vi "PRO_VerifySpec.vi"(6 "error in (no error)":errorcluster, 7 "Enable":bool, 8 "Results in":T6=[[{"Fill"=0.0, "Drain"=7.150000000000002, "Status"=9, "Resistor"=100.0}, {"Fill"=0.0, "Drain"=6.925000000000003, "Status"=9, "Resistor"=100.0}], [{"Fill"=7.1350000000000025, "Drain"=6.700000000000004, "Status"=9, "Resistor"=200.0}, {"Fill"=6.910000000000004, "Drain"=6.475000000000005, "Status"=9, "Resistor"=200.0}], [{"Fill"=6.685000000000004, "Drain"=6.250000000000005, "Status"=9, "Resistor"=300.0}, {"Fill"=6.460000000000004, "Drain"=6.025000000000006, "Status"=9, "Resistor"=300.0}], [{"Fill"=6.235000000000006, "Drain"=5.8000000000000025, "Status"=9, "Resistor"=400.0}, {"Fill"=6.010000000000005, "Drain"=5.59, "Status"=9, "Resistor"=400.0}], [{"Fill"=5.785000000000002, "Drain"=5.364999999999997, "Status"=9, "Resistor"=500.0}, {"Fill"=5.574999999999999, "Drain"=5.1399999999999935, "Status"=9, "Resistor"=500.0}], [{"Fill"=5.349999999999996, "Drain"=4.91499999999999, "Status"=9, "Resistor"=600.0}, {"Fill"=5.124999999999993, "Drain"=4.689999999999987, "Status"=9, "Resistor"=600.0}], [{"Fill"=4.89999999999999, "Drain"=4.464999999999983, "Status"=9, "Resistor"=700.0}, {"Fill"=4.6749999999999865, "Drain"=4.23999999999998, "Status"=9, "Resistor"=700.0}], [{"Fill"=4.449999999999983, "Drain"=4.014999999999977, "Status"=9, "Resistor"=800.0}, {"Fill"=4.22499999999998, "Drain"=3.7899999999999734, "Status"=9, "Resistor"=800.0}], [{"Fill"=3.999999999999977, "Drain"=3.56499999999997, "Status"=9, "Resistor"=900.0}, {"Fill"=3.7749999999999737, "Drain"=3.339999999999967, "Status"=9, "Resistor"=900.0}], [{"Fill"=3.5499999999999705, "Drain"=3.114999999999964, "Status"=9, "Resistor"=1000.0}, {"Fill"=3.3249999999999673, "Drain"=2.8899999999999606, "Status"=9, "Resistor"=1000.0}], [{"Fill"=3.099999999999964, "Drain"=0.0, "Status"=5, "Resistor"=1100.0}, {"Fill"=2.874999999999961, "Drain"=0.0, "Status"=5, "Resistor"=1100.0}]] {"Resistor" format="%.1f"; "Drain" format="%.3f"; "Fill" format="%.3f"}, 9 "Measure In":T5={"Ch A   Ohms"=100.0, " Ch B  Ohms"=100.0, "Level OUt"=3.672222222222213}, 10 "Specs In":T1) -> (0 "Results out":T6=[[{"Fill"=0.0, "Drain"=7.150000000000002, "Status"=9, "Resistor"=100.0}, {"Fill"=0.0, "Drain"=6.925000000000003, "Status"=9, "Resistor"=100.0}], [{"Fill"=7.1350000000000025, "Drain"=6.700000000000004, "Status"=9, "Resistor"=200.0}, {"Fill"=6.910000000000004, "Drain"=6.475000000000005, "Status"=9, "Resistor"=200.0}], [{"Fill"=6.685000000000004, "Drain"=6.250000000000005, "Status"=9, "Resistor"=300.0}, {"Fill"=6.460000000000004, "Drain"=6.025000000000006, "Status"=9, "Resistor"=300.0}], [{"Fill"=6.235000000000006, "Drain"=5.8000000000000025, "Status"=9, "Resistor"=400.0}, {"Fill"=6.010000000000005, "Drain"=5.59, "Status"=9, "Resistor"=400.0}], [{"Fill"=5.785000000000002, "Drain"=5.364999999999997, "Status"=9, "Resistor"=500.0}, {"Fill"=5.574999999999999, "Drain"=5.1399999999999935, "Status"=9, "Resistor"=500.0}], [{"Fill"=5.349999999999996, "Drain"=4.91499999999999, "Status"=9, "Resistor"=600.0}, {"Fill"=5.124999999999993, "Drain"=4.689999999999987, "Status"=9, "Resistor"=600.0}], [{"Fill"=4.89999999999999, "Drain"=4.464999999999983, "Status"=9, "Resistor"=700.0}, {"Fill"=4.6749999999999865, "Drain"=4.23999999999998, "Status"=9, "Resistor"=700.0}], [{"Fill"=4.449999999999983, "Drain"=4.014999999999977, "Status"=9, "Resistor"=800.0}, {"Fill"=4.22499999999998, "Drain"=3.7899999999999734, "Status"=9, "Resistor"=800.0}], [{"Fill"=3.999999999999977, "Drain"=3.56499999999997, "Status"=9, "Resistor"=900.0}, {"Fill"=3.7749999999999737, "Drain"=3.339999999999967, "Status"=9, "Resistor"=900.0}], [{"Fill"=3.5499999999999705, "Drain"=3.114999999999964, "Status"=9, "Resistor"=1000.0}, {"Fill"=3.3249999999999673, "Drain"=2.8899999999999606, "Status"=9, "Resistor"=1000.0}], [{"Fill"=3.099999999999964, "Drain"=0.0, "Status"=5, "Resistor"=1100.0}, {"Fill"=2.874999999999961, "Drain"=0.0, "Status"=5, "Resistor"=1100.0}]] {"Resistor" format="%.1f"; "Drain" format="%.3f"; "Fill" format="%.3f"}, 1 "Status Code":i32, 4 "error out":errorcluster)   [LabVIEW 2024]
doc: "Compares the ChA, ChB and Level measurements to the Incexed Spec Row. Checks for R Switch Value occured in Switch Zone, The resistor level was consistand in the In Range Zone, and records the R level in ohms at the R measurement point. \n\nBuilds the Results Table."
uses:
  Control Definitions/Def Results2.ctl
  Control Definitions/DEF_SpecsOut.ctl
  Control Definitions/Ded Spec RNG.ctl
  Control Definitions/Ded LUT_Status.ctl
  Control Definitions/Def PumpCtlRefs.ctl
panel:
  # "ChA=0; ChB=1"
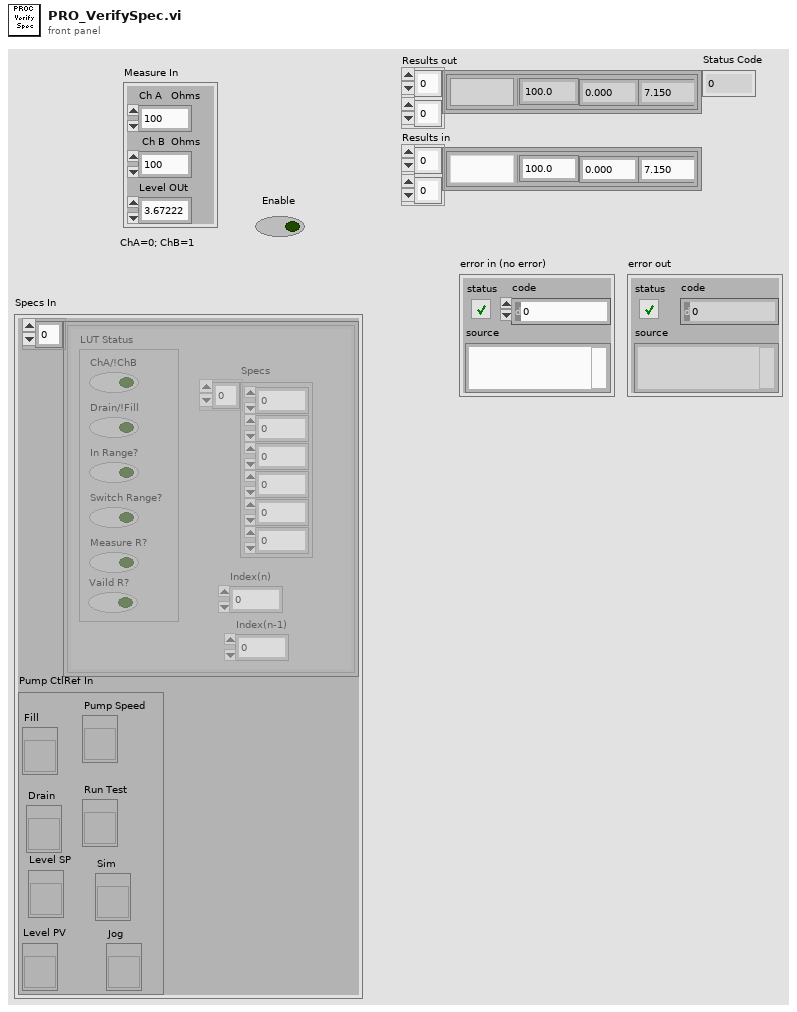
[diagram p1: front panel]
types:
  T1 = typedef "DEF_SpecsOut.ctl" = cluster{"aSpecsTable":T2[], "Pump CtlRef In":T4}
  T2 = typedef "Ded Spec RNG.ctl" = cluster{"Specs":dbl[], "Index(n)":i32, "LUT Status":T3, "Index(n-1)":i32}
  T3 = typedef "Ded LUT_Status.ctl" = cluster{"ChA/!ChB":bool, "Drain/!Fill":bool, "In Range?":bool, "Switch Range?":bool, "Measure R?":bool, "Vaild R?":bool}
  T4 = typedef "Def PumpCtlRefs.ctl" = cluster{"Fill ":refnum<vi>, "Drain":refnum<vi>, "Level PV":refnum<vi>, "Pump Speed":refnum<vi>, "Run Test":refnum<vi>, "Sim":refnum<vi>, "Jog":refnum<vi>, "Level SP":refnum<vi>}
  T5 = cluster{"Ch A   Ohms":dbl, " Ch B  Ohms":dbl, "Level OUt":dbl}
  T6 = typedef "Def Results2.ctl" = cluster{"Fill":dbl, "Drain":dbl, "Status":i16, "Resistor":dbl}[][]
  T7 = cluster{"Fill":dbl, "Drain":dbl, "Status":i16, "Resistor":dbl}
  T8 = typedef "Def_LevelSwitched.ctl" = cluster{"Switched":bool, "Level OUt":dbl}
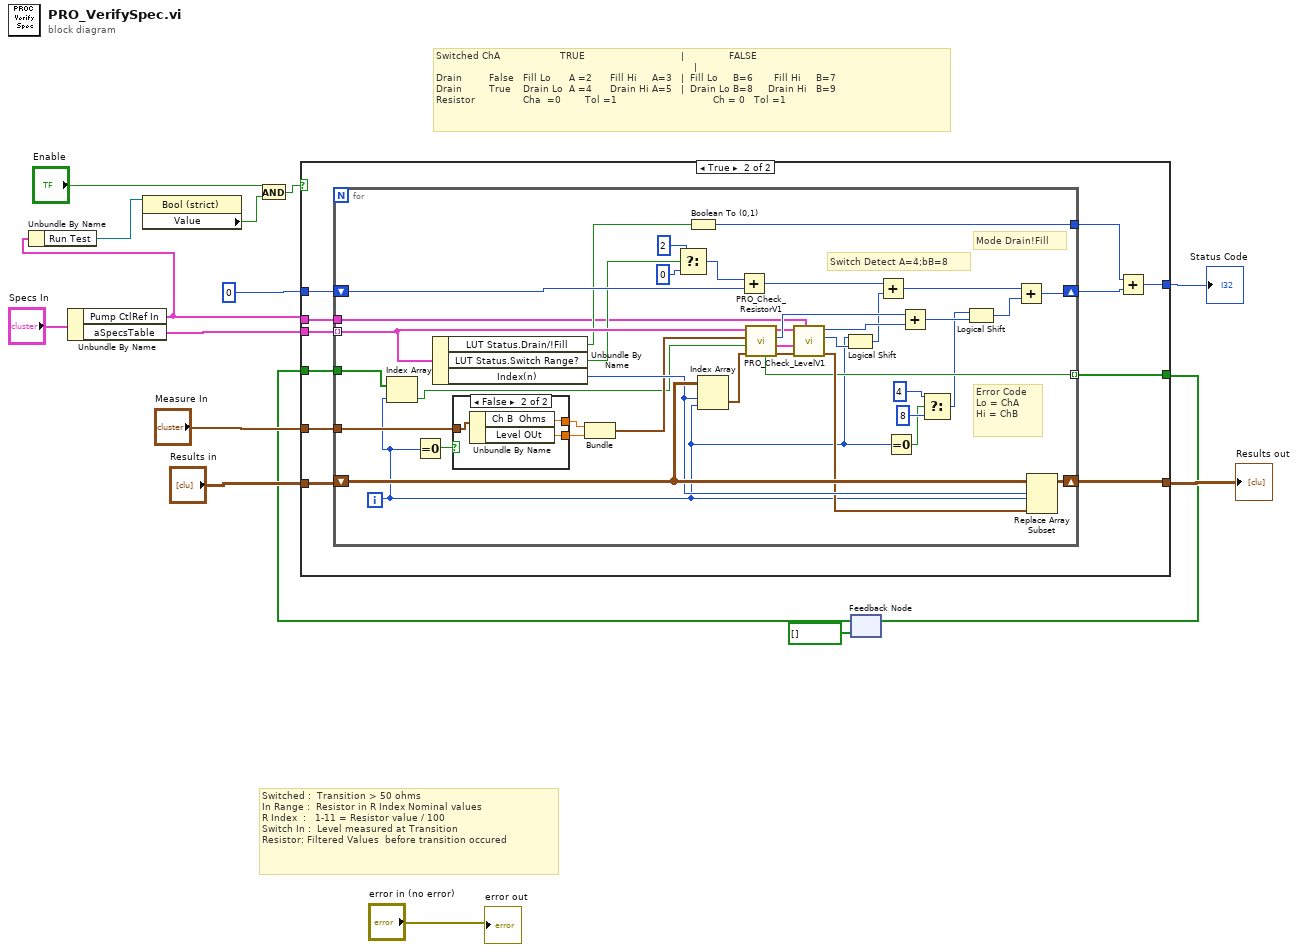
[diagram p0: block diagram]
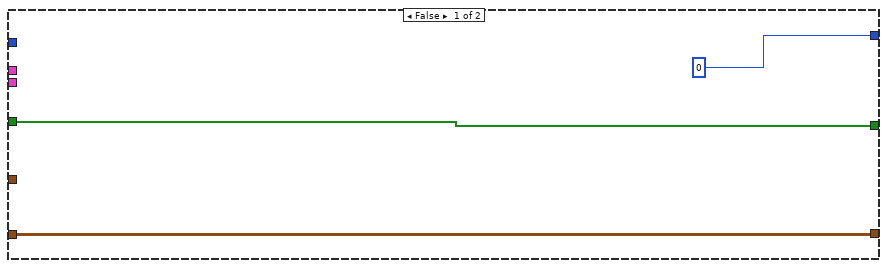
[diagram p2: hidden frame]
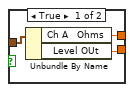
[diagram p3: hidden frame]
diagram:
  # "Switched ChA                    TRUE                                |               FALSE\n                                                                                      |\nDrain         False   Fill Lo      A =2      Fill Hi     A=3   |  Fill Lo     B=6       Fill Hi     B=7\nDrain         True    Drain Lo  A =4      Drain Hi A=5   |  Drain Lo B=8     Drain Hi   B=9 \nResistor                Cha  =0        Tol =1                                Ch = 0   Tol =1"
  # "Switched :  Transition > 50 ohms\nIn Range :  Resistor in R Index Nominal values\nR Index  :   1-11 = Resistor value / 100\nSwitch In :  Level measured at Transition\nResistor: Filtered Values  before transition occured"
  n1 = Unbundle By Name("Specs In") -> ("Pump CtlRef In"=w8:T4, "aSpecsTable"=w9:T2[])
  n2 = Unbundle By Name(w8) -> ("Run Test"=w7:refnum<vi>)
  n3 = property class="Bool (strict)"(reference=w7) -> ("Value"=w5:bool)  [unwired: 1 in, 2 out]
  n4 = And(x="Enable", y=w5) -> (x .and. y?=w6:bool)
  n5 = feedback #1(bool[] []) -> (w2:bool[])
  n6 = case shown="True" w6 {
    tunnel: w9 -> [_ w30]
    tunnel: "Results in" -> [w18 w29]
    tunnel: [w18 w28] -> w14
    tunnel: 0 -> [_ w27]
    tunnel: [0 w23] -> w12
    tunnel: "Measure In" -> [_ w26]
    tunnel: w2 -> [w17 w24]
    tunnel: [w17 w25] -> w3
    tunnel: w8 -> [_ w20]
    frame False {
    }
    frame True {
      n7 = for {
        tunnel: w30 -> [w63] mode=indexing
        shift-right: [w53] -> w28
        shift-left: w29 -> [w69]
        shift-right: [w50] -> w22
        shift-left: w27 -> [w44]
        tunnel: w26 -> [w66]
        tunnel: [w52] -> w25 mode=indexing
        tunnel: w24 -> [w56]
        tunnel: [w35] -> w21
        tunnel: w20 -> [w31]
        i -> [w41]
        # "Switch Detect A=4;bB=8"
        # "Mode Drain!Fill"
        # "Error Code\nLo = ChA\nHi = ChB"
        n8 = Index Array(array=w56, index=w41) -> (element=w32:bool)
        n9 = Equal To 0?(x=w41) -> (x = 0?=w65:bool)
        n10 = Unbundle By Name(w63) -> ("LUT Status.Drain/!Fill"=w37:bool, "LUT Status.Switch Range?"=w34:bool, "Index(n)"=w68:i32)
        n11 = case shown="False" w65 {
          tunnel: w66 -> [w72 w75]
          tunnel: [w71 w74] -> w64
          tunnel: [w70 w73] -> w33
          frame True {
            n12 = Unbundle By Name(w72) -> ("Ch A   Ohms"=w71:dbl, "Level OUt"=w70:dbl)
          }
          frame False {
            n13 = Unbundle By Name(w75) -> ("Ch B  Ohms"=w74:dbl, "Level OUt"=w73:dbl)
          }
        }
        n14 = Bundle("Ch B  Ohms"=w64, "Level OUt"=w33) -> (w62:cluster{" Ch B  Ohms":dbl, "Level OUt":dbl})  [unwired: 1 in]
        n15 = Select(t=2, s=w34, f=0) -> (s? t:f=w36:i32)
        n16 = Boolean To (0,1)(Boolean=w37) -> (0, 1=w35:i16)
        n17 = Index Array(array=w69, index (row)=w68, index (col)=w41) -> (element=w61:T7)
        n18 = Add(x=w36, y=w44) -> (x+y=w43:i32)
        n19 = call "PRO_Check_ResistorV1.vi"("Results In"=w61, "Switched In"=w32, "Inputs"=w62, "ChA Spec RNG In"=w63) -> ("Results out"=w59:T7, "Level Out"=w58:T8, "Err Num"=w60:i32, "ChA Spec RNG Out"=w57:T2, "Switched Out"=w52:bool)  [unwired: 3 in]
        n20 = call "PRO_Check_LevelV1.vi"("cluster"=w31, "Results in"=w59, "Level In"=w58, "ChA Spec RNG In"=w57) -> ("Results out"=w67:T7, "Switched Code"=w42:i32, "Err Num"=w46:i32)  [unwired: 4 in, 1 out]
        n21 = Logical Shift(y=w41, x=w42) -> (x << y=w45:i32)
        n22 = Add(x=w43, y=w45) -> (x+y=w38:i32)
        n23 = Equal To 0?(x=w41) -> (x = 0?=w51:bool)
        n24 = Add(x=w60, y=w46) -> (x+y=w40:i32)
        n25 = Select(t=4, s=w51, f=8 ("x")) -> (s? t:f=w39:i32)
        n26 = Logical Shift(y=w39, x=w40) -> (x << y=w47:i32)
        n27 = Add(x=w38, y=w47) -> (x+y=w50:i32)
        n28 = Replace Array Subset(array=w69, new element=w67, index (row)=w68, index (col)=w41) -> (w53:T6)
      }
      n29 = Add(x=w21, y=w22) -> (x+y=w23:i32)
    }
  }
  "Results out" <- w14
  "Status Code" <- w12
  n30 = feedback-in #1(w3) -> ()
  "error out" <- "error in (no error)"
